vi "UART Init Device.vi"(8 "error in (no error)":errorcluster, 9 "pInitConfig":T1, 10 "UARTIndex":i32, 11 "DevIndex":i32) -> (0 "error out":errorcluster, 3 "function return":i32)   [LabVIEW 2012, in "ControlUART.lvlib"]
doc: "int WINAPI UART_InitDevice(int DevIndex,int UARTIndex, PUART_INIT_CONFIG pInitConfig);"
uses:
  ControlUART.lvlib
  Ginkgo_Driver.dll
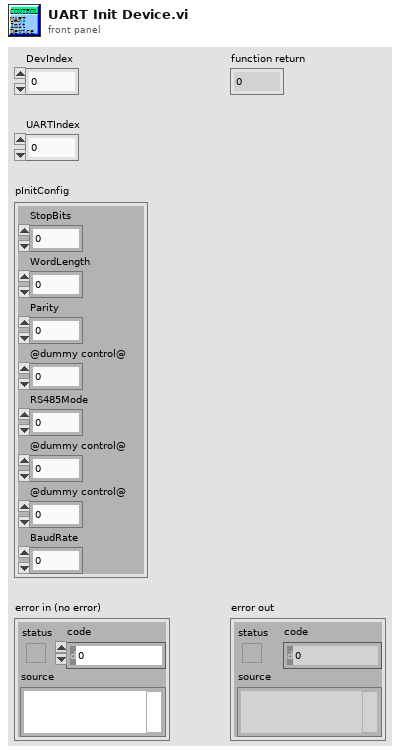
[diagram p1: front panel]
types:
  T1 = cluster{"StopBits":u8, "WordLength":u8, "Parity":u8, "@dummy control@":i8, "RS485Mode":u16, "@dummy control@":i8, "@dummy control@":i8, "BaudRate":u32}
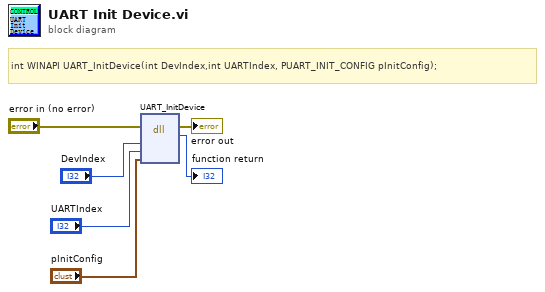
[diagram p0: block diagram]
diagram:
  # "int WINAPI UART_InitDevice(int DevIndex,int UARTIndex, PUART_INIT_CONFIG pInitConfig);"
  n1 = dll-call lib="E:/Project/vt_ginkgo/truck/Ginkgo Driver/vs2010/Ginkgo_USB-I2C_API_v2.0.3.0/lib/labview_32bit/ControlUART/Ginkgo_Driver.*" fn="UART_InitDevice"(error in="error in (no error)", "DevIndex"="DevIndex", "UARTIndex"="UARTIndex", "pInitConfig"="pInitConfig") -> (error out=→"error out":errorcluster, →"function return":i32)  [unwired: 5 in, 1 out]
